vi "ModBus_CRC.vi"(8 "error in (no error)":errorcluster, 11 "string in":string) -> (0 "error out":errorcluster, 3 "String + CRC":string)   [LabVIEW 2018]
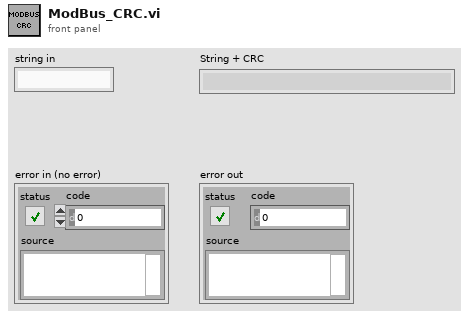
[diagram p1: front panel]
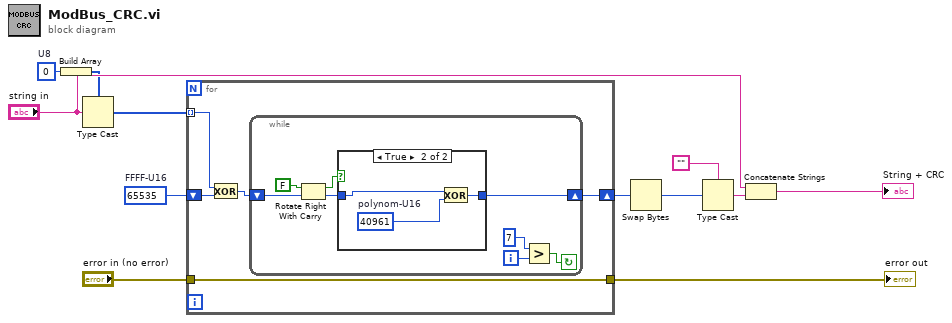
[diagram p0: block diagram]
diagram:
  w7 = u16 65535  # FFFF-U16
  w4 = u8 0  # U8
  n1 = Build Array(w4) -> (w5:u8[])
  n2 = Type Cast(type=w5, x="string in") -> (*(type *) &x=w6:u8[])
  n3 = for {
    tunnel: w6 -> [w16] mode=indexing
    shift-right: [w14] -> w8
    shift-left: w7 -> [w17]
    tunnel: "error in (no error)" -> [w13]
    tunnel: [w13] -> w1
    n4 = Exclusive Or(1:w17, 2:w16) -> (0:w15:u16)
    n5 = while {
      shift-right: [w18] -> w14
      shift-left: w15 -> [w25]
      i -> [w21]
      stop <- w22 continue-if-true
      n6 = Rotate Right With Carry(2:w25, 3:FALSE ("carry")) -> (0:w19:u16, 1:w24:bool)
      n7 = case shown="True" w24 {
        tunnel: w19 -> [w26 w29]
        tunnel: [w26 w28] -> w18
        frame False {
        }
        frame True {
          w27 = u16 40961  # polynom-U16
          n8 = Exclusive Or(1:w27, 2:w29) -> (0:w28:u16)
        }
      }
      n9 = Greater?(x=7, y=w21) -> (0:w22:bool)
    }
  }
  "error out" <- w1
  n10 = Swap Bytes(anything=w8) -> (byte swapped=w11:u16)
  n11 = Type Cast(type="", x=w11) -> (*(type *) &x=w10:string)
  n12 = Concatenate Strings("string in", w10) -> (→"String + CRC":string)
